vi "findnextfilenum.vi"(6 "digits":dbl, 7 "extension":string, 8 "filename":string, 9 "Path":path) -> (2 "Output":dbl, 3 "fulloutputpath":path)   [LabVIEW 2009]
panel:
  out "String 2":string
  out "Output 2":dbl
  out "String":string
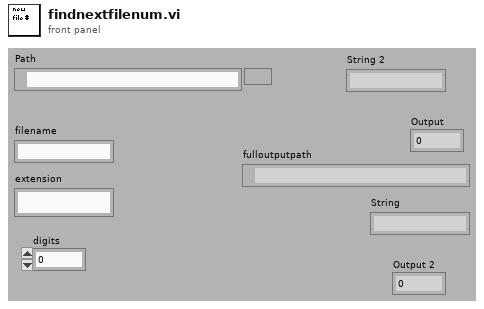
[diagram p1: front panel]
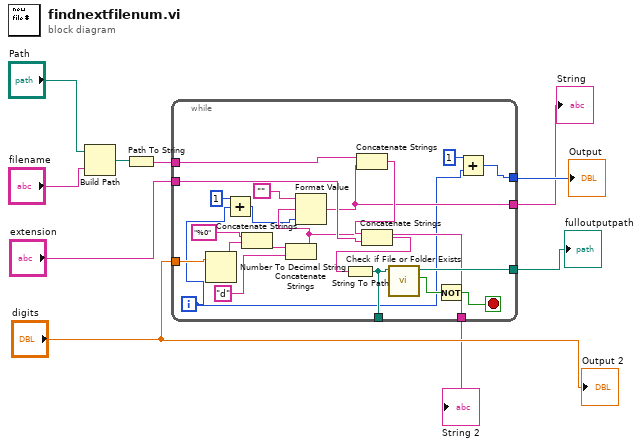
[diagram p0: block diagram]
diagram:
  n1 = Build Path(base path="Path", name or relative path="filename") -> (appended path=w3:path)
  n2 = Path To String(path=w3) -> (string=w4:string)
  n3 = while {
    tunnel: w4 -> [w31]
    tunnel: "extension" -> [w30]
    tunnel: "digits" -> [w20]
    tunnel: [w27] -> w9
    tunnel: [w11] -> w8
    tunnel: [w21] -> w7
    tunnel: [w19] -> w5
    tunnel: [w16] -> _
    i -> [w13]
    stop <- w25 stop-if-true
    n4 = Number To Decimal String(number=w20) -> (decimal integer string=w17:string)  [unwired: 1 in]
    n5 = Add(x=1, y=w13) -> (x+y=w14:i32)
    n6 = Concatenate Strings("%0", w17) -> (w23:string)
    n7 = Concatenate Strings(w23, "d") -> (w19:string)
    n8 = Format Value(string ("")="", format string=w19, value (0)=w14) -> (output string=w21:string)
    n9 = Concatenate Strings(w31, w21) -> (w29:string)
    n10 = Concatenate Strings(w29, w30) -> (w28:string)
    n11 = String To Path(string=w28) -> (path=w16:path)
    n12 = call <vilib>:"Check if File or Folder Exists.vi"("path"=w16) -> ("file or folder exists?"=w26:bool, "dup path"=w27:path)  [unwired: 8 in, 1 out]
    n13 = Not(x=w26) -> (.not. x?=w25:bool)
    n14 = Add(x=1, y=w13) -> (x+y=w11:i32)
  }
  "Output" <- w8
  "fulloutputpath" <- w9
  "String" <- w7
  "String 2" <- w5
  "Output 2" <- "digits"
